vi "PlotMieCurveFromRICheckMieFunction.vi"(1 "max size parameter alpha\n(alpha = 2Pi*r/lambda)":sgl=20.0 step=0.01 format="%.2f", 2 "refractive index, imaginary":dbl step=0.009999999776482582 format="%.4f", 3 "refractive index, real":sgl=1.3 step=0.01 format="%.4f") -> (0 "Extinction Graph":cluster{"Signal":dbl[], "Signal":dbl[]}[](graph))   [LabVIEW 2011]
uses:
  <vilib>/Platform/storage/lvStorage.llb/_openFunction.ctl
  <vilib>/Analysis/1siggen.llb/Ramp Pattern by Samples.vi
  <vilib>/Platform/storage/lvStorage.llb/_defaultFilePath.vi
  <vilib>/Platform/storage/lvStorage.llb/_openStorageWithRootAutoDetect.vi
  <vilib>/Platform/storage/lvStorage.llb/xStorage/xStorageSupp/ErrorOut.vi
  <vilib>/Platform/storage/lvStorage.llb/_queryPropDateTime.vi
  <vilib>/Platform/storage/lvStorage.llb/_queryGenericObjects.vi
  <vilib>/Platform/storage/lvStorage.llb/_loadAllDouble.vi
  <vilib>/Platform/storage/Storage.llb/Get Object Info.vi
  <vilib>/Platform/storage/Storage.llb/__closeStorageFromObject.vi
  <vilib>/Platform/storage/lvStorage.llb/xStorage/Open Data Storage/Open Data Storage.xnode
  <vilib>/Platform/storage/lvStorage.llb/xStorage/Read Data/Read Data.xnode
  <vilib>/Platform/storage/lvStorage.llb/xStorage/Close Data Storage/Close Data Storage.xnode
  mie2.dll
  <vilib>/Analysis/NI_AALBase.lvlib
panel:
  out "Ramp Pattern":dbl[](array[numeric])
  out "subarray":dbl[](array[numeric])
  out "x-y":dbl[](array[numeric])
  out "Extinction Graph 2":cluster{"Ramp Pattern":dbl[], dbl[]}(graph)
  in  "file path":path
  in  "Number of particle sizes for expected values":i32=1000
  out "totalscatter":sgl=2.73535
  out "backscatter":sgl=1.1527499
  out "<cos(theta)> 2":sgl=0.84980327
  out "extinction":sgl=2.7353504
  in  "angles (will compute\n2*angles-1 points from\n0...180 degrees)":u32=2
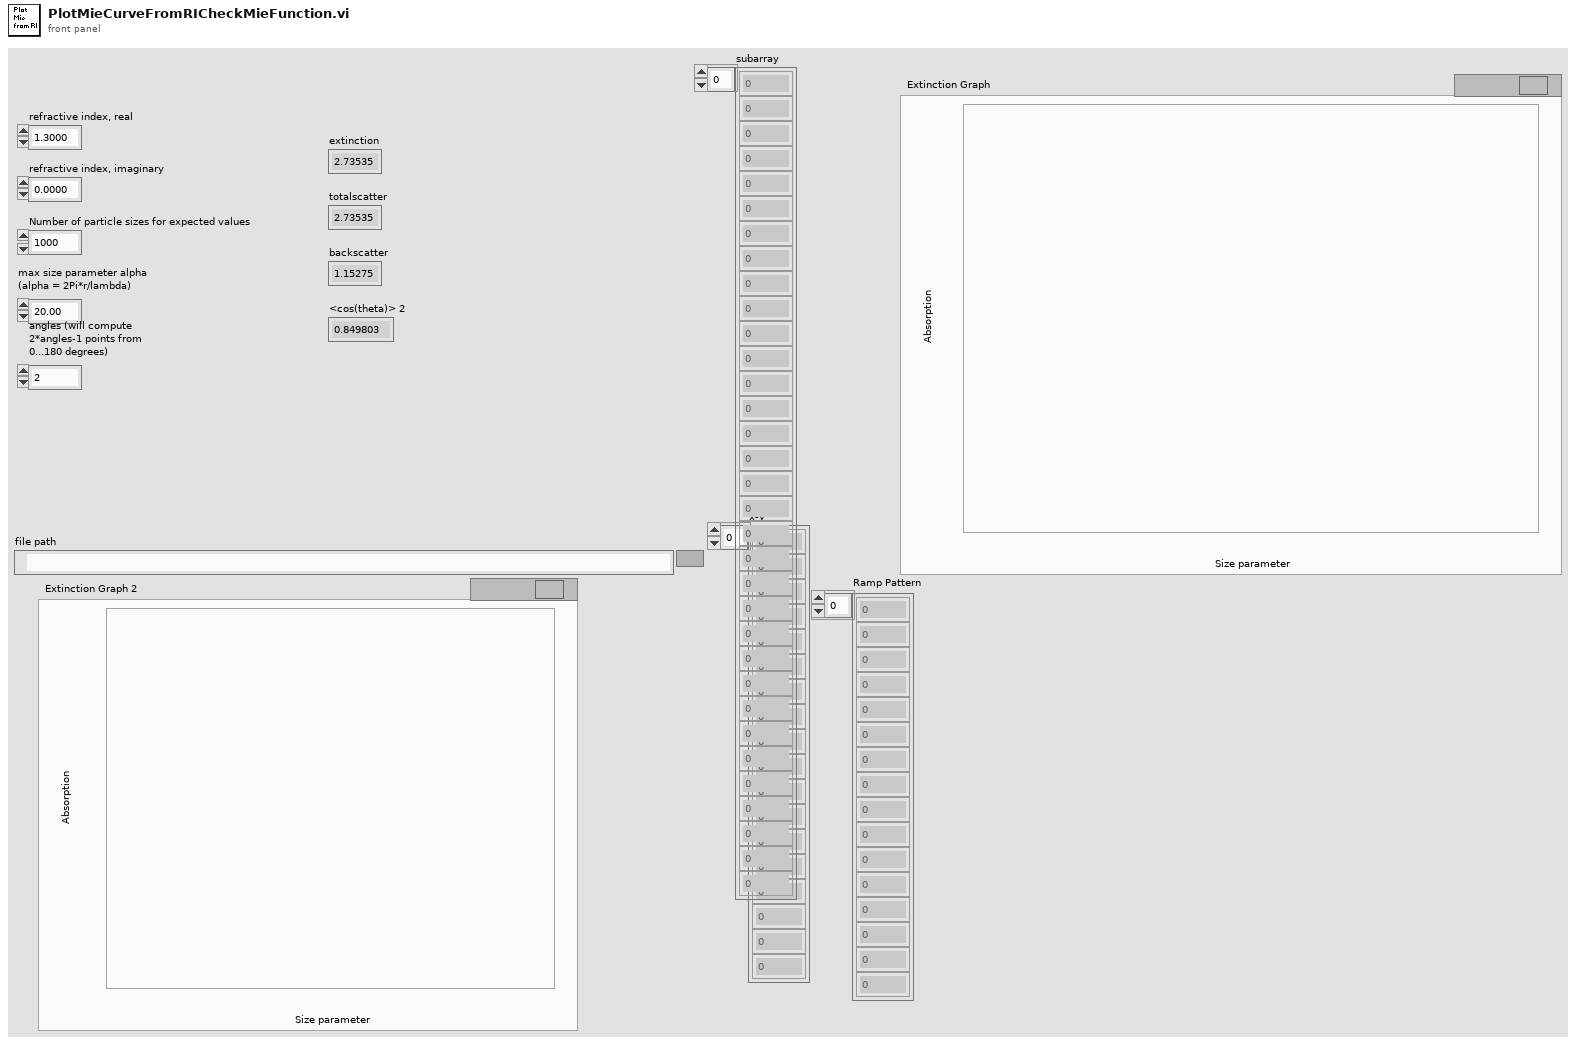
[diagram p1: front panel]
types:
  T1 = enum16{"open", "open or create", "create or replace", "create", "open (read only)"}
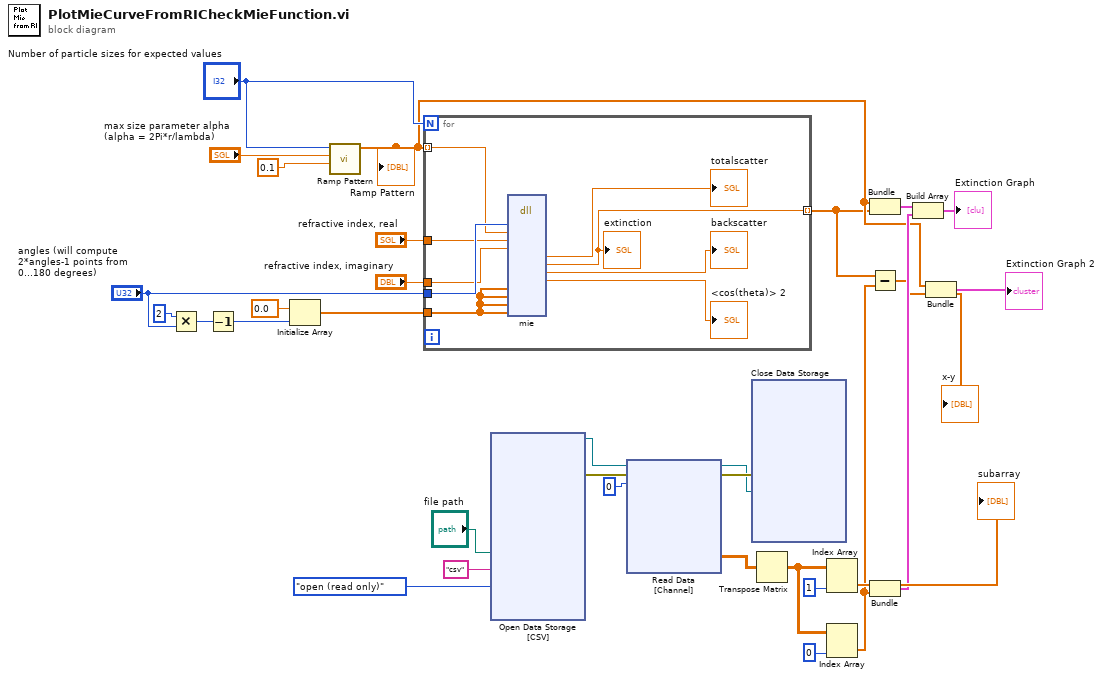
[diagram p0: block diagram]
diagram:
  n1 = Multiply(x=u32 2, y="angles (will compute\n2*angles-1 points from\n0...180 degrees)") -> (x*y=w31:u32)
  n2 = Decrement(x=w31) -> (x-1=w29:u32)
  n3 = Initialize Array(sgl 0.0, w29) -> (w23:sgl[])
  n4 = call-poly <vilib>:"Ramp Pattern.vi"("start"=0.1, "end"="max size parameter alpha\n(alpha = 2Pi*r/lambda)", "samples"="Number of particle sizes for expected values") -> ("Ramp Pattern"=w5:dbl[])  [unwired: 7 in, 1 out]
  "Ramp Pattern" <- w5
  n5 = for {
    N: "Number of particle sizes for expected values" -> [_]
    tunnel: w23 -> [w39]
    tunnel: "angles (will compute\n2*angles-1 points from\n0...180 degrees)" -> [w38]
    tunnel: "refractive index, real" -> [w37]
    tunnel: "refractive index, imaginary" -> [w36]
    tunnel: w5 -> [w34] mode=indexing
    tunnel: [w33] -> w4 mode=indexing
    n6 = dll-call lib="Z:/Dropbox/Lior Segev/Lior Segev Projects/RI retrieval in Labview/RIRetrievalInLabViewVer2/mie2.dll" fn="mie"("angles"=w38, "x"=w34, "r"=w37, "i"=w36, "spol_real"=w39, "spol_imaginary"=w39, "ppol_real"=w39, "ppol_imaginary"=w39) -> ("totalscatter"=→"totalscatter":sgl, "extinction"=w33:sgl, "backscatter"=→"backscatter":sgl, "<cos(theta)>"=→"<cos(theta)> 2":sgl)  [unwired: 16 in, 2 out]
    "extinction" <- w33
  }
  n7 = xnode "Open Data Storage\n[CSV]"("file path"="file path", "DataPlugin name"="csv", "function (open:0)"=T1."open (read only)") -> ("storage refnum (file)"=w21:refnum<k20>, "error out"=w20:errorcluster)  [unwired: 2 in, 1 out]
  n8 = xnode "Read Data\n[Channel]"("storage refnum (file)"=w21, "error in"=w20, "index"=0) -> ("Signal"=w13:dbl[][], "storage refnum (file) out"=w16:refnum<k20>, "error out"=w19:errorcluster)  [unwired: 1 in, 1 out]
  n9 = xnode "Close Data Storage\n"("error in (no error)"=w19, "storage refnum (file)"=w16) -> ()  [unwired: 2 out]
  n10 = Transpose Matrix(1:w13) -> (0:w11:dbl[][])
  n11 = Index Array(array=w11, index (col)=1 ("disabled index (col)")) -> (element=w9:dbl[])  [unwired: 1 in]
  "subarray" <- w9
  n12 = Index Array(array=w11, index (col)=0 ("disabled index (col)")) -> (element=w3:dbl[])  [unwired: 1 in]
  n13 = Bundle("Ramp Pattern"=w5, w4) -> (w7:cluster{"Ramp Pattern":dbl[], sgl[]})  [unwired: 1 in]
  n14 = Subtract(x=w4, y=w3) -> (x-y=w2:dbl[])
  "x-y" <- w2
  n15 = Bundle("Signal"=w9, "Signal"=w3) -> (w6:cluster{"Signal":dbl[], "Signal":dbl[]})  [unwired: 1 in]
  n16 = Build Array(w7, w6) -> (→"Extinction Graph":cluster{"Signal":dbl[], "Signal":dbl[]}[])
  n17 = Bundle("Ramp Pattern"=w5, w2) -> (→"Extinction Graph 2":cluster{"Ramp Pattern":dbl[], dbl[]})  [unwired: 1 in]
